vi "previewMovingBallIntercept.vi"(7 "destino original":dbl[](array[numeric]), 8 "error in (no error)":errorcluster, 9 "Robot in":refnum<class "Robot.lvclass">, 10 "BallRef":refnum<class "Ball.lvclass">, 11 "KickToSkill in":refnum<class "KickToSkill.lvclass">) -> (0 "error out":errorcluster, 1 "estimated_intercep_point":dbl[](array[numeric]), 2 "heuristic":dbl, 3 "KickToSkill out":refnum<class "KickToSkill.lvclass">)   [LabVIEW 2023, in "KickToSkill.lvclass"]
uses:
  KickToSkill.lvclass
  Robot_class/Robot.lvclass
  C:/Users/ebert/Documents/codes/SSL/repo/SSL_AI/Object_class/Object.lvclass
  Ball_class/Ball.lvclass
  Object_class/Object.lvclass/Object.ctl
  Ball_class/Ball.lvclass/Ball.ctl
  <vilib>/Analysis/baseanly.llb/Unit Vector (DBL).vi
  <vilib>/Analysis/_algsub.llb/Real Vector Norm.vi
  Object_class/Read x.vi
  Object_class/Read y.vi
  Ball_class/Read v_x.vi
  Ball_class/Read v_y.vi
  KickToSkill.lvclass/KickToSkill.ctl
  <vilib>/Analysis/NI_AALPro.lvlib
  <vilib>/Analysis/NI_AALBase.lvlib
  Game_class/Game.lvclass
  <vilib>/Analysis/baseanly.llb/Real Dot Product.vi
panel:
  out "Waveform Chart":dbl(graph)
  out "Array":dbl[][](array[numeric])
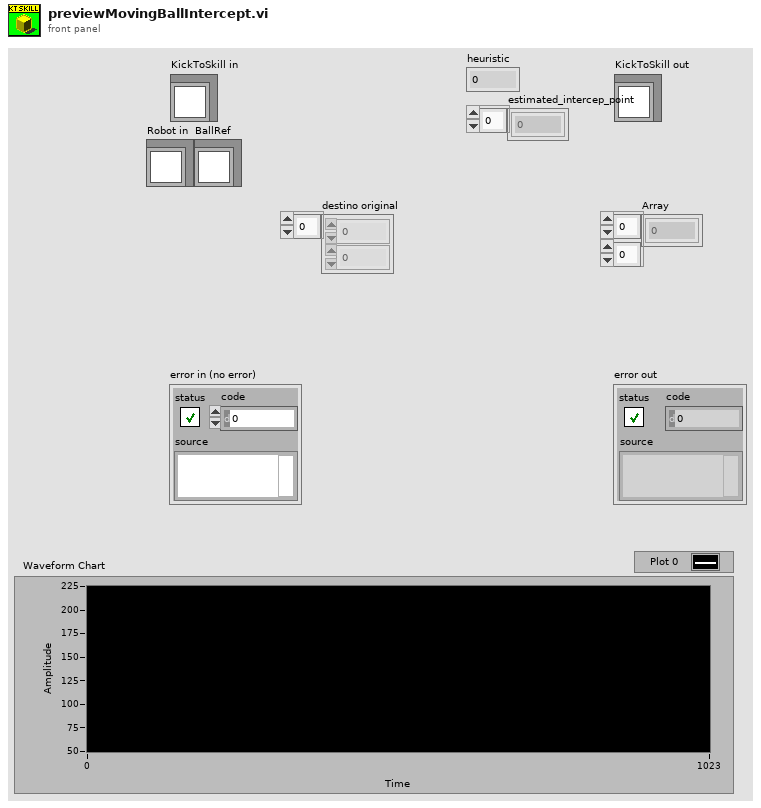
[diagram p1: front panel]
types:
  T1 = typedef "NI_Matrix.lvlib/RealMatrix.ctl" = dbl[][]
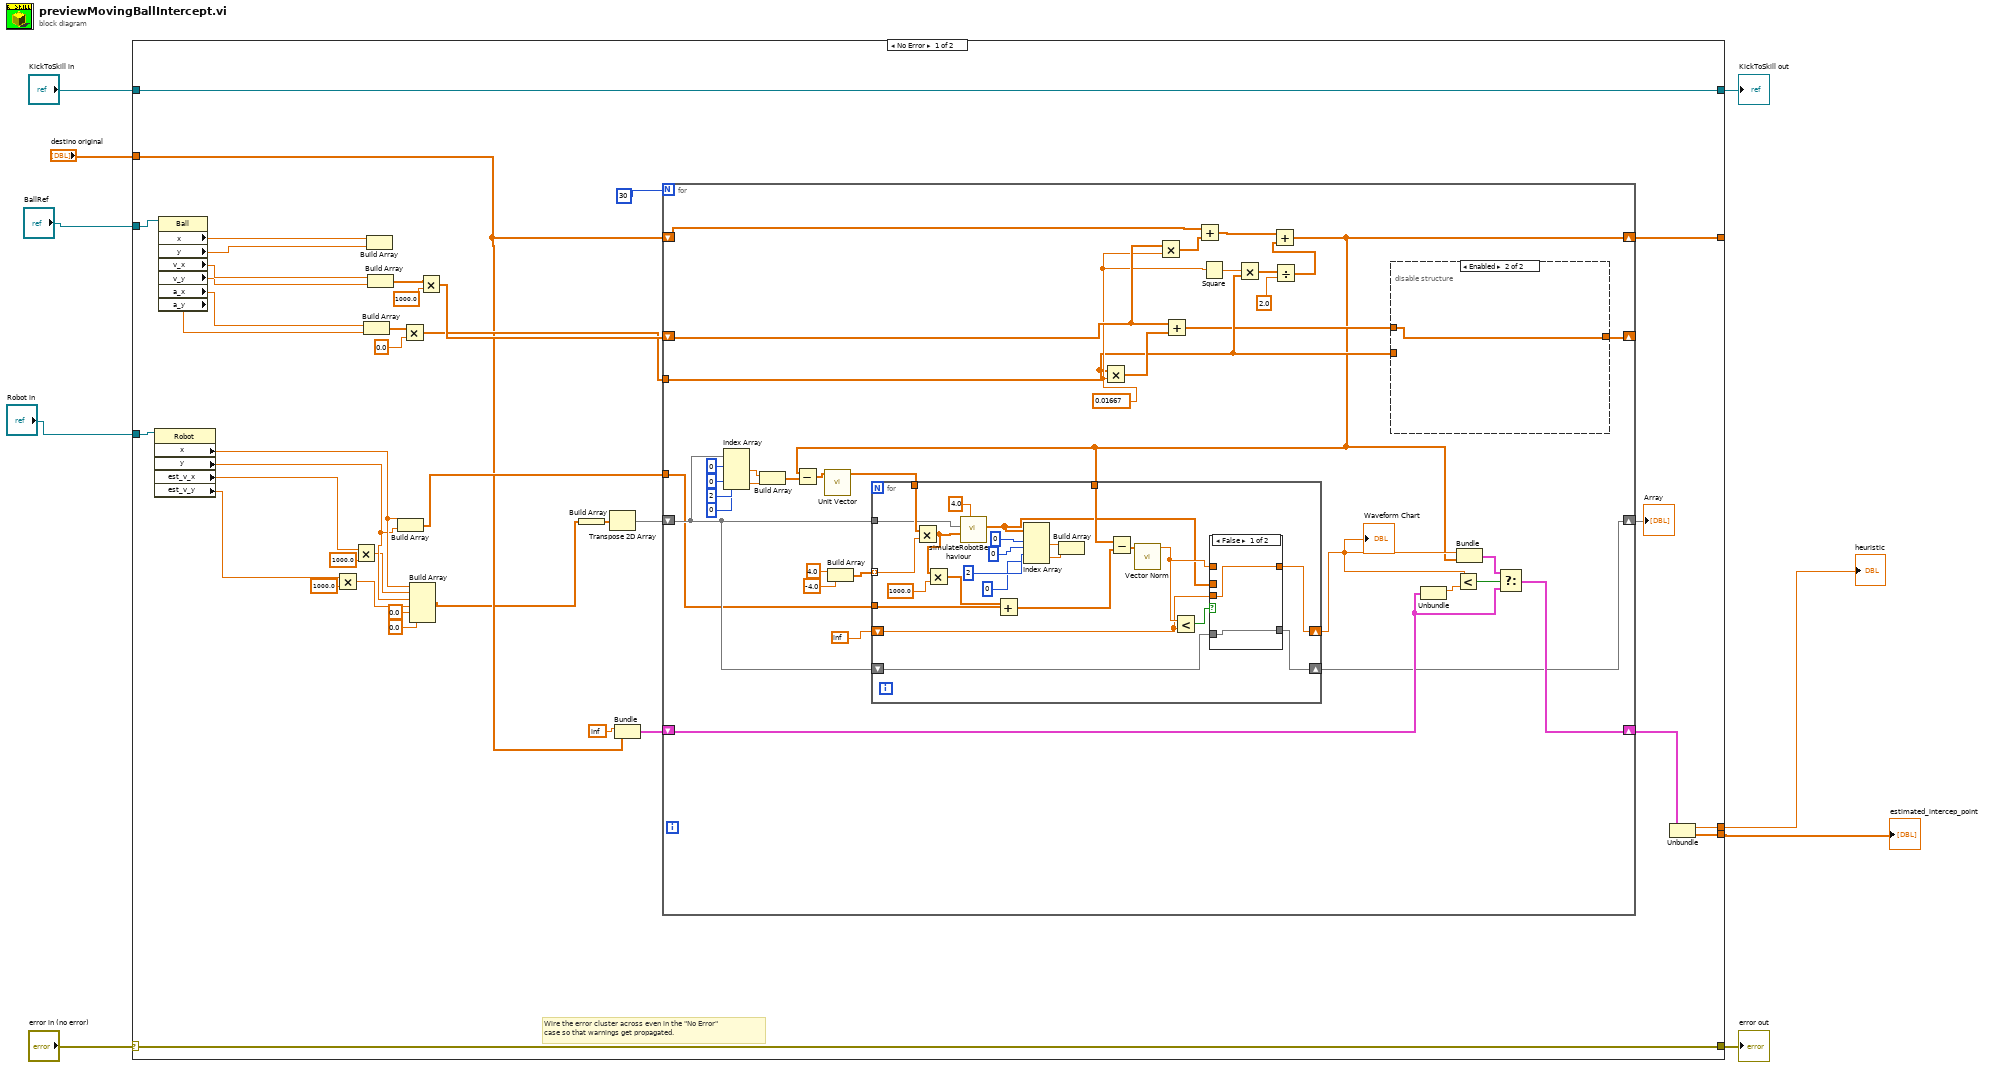
[diagram p0: block diagram]
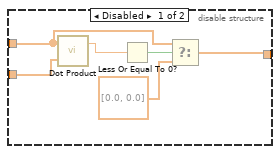
[diagram p3: hidden frame]
diagram:
  n1 = case shown="No Error" "error in (no error)" {
    selector: "error in (no error)" -> [w47 w121]
    tunnel: [w47 w121] -> w8
    tunnel: [w48 w120] -> w6
    tunnel: "KickToSkill in" -> [w48 w120]
    tunnel: "BallRef" -> [w44 _]
    tunnel: "Robot in" -> [w39 _]
    tunnel: [w36 _] -> w5
    tunnel: [w10 _] -> w4
    tunnel: [w11 _] -> _
    tunnel: "destino original" -> [w21 _]
    frame No Error {
      # "Wire the error cluster across even in the \"No Error\"\ncase so that warnings get propagated."
      n2 = property class="Robot"(reference=w39) -> ("x"=w27:dbl, "y"=w26:dbl, "est_v_x"=w16:dbl, "est_v_y"=w14:dbl)  [unwired: 1 in, 2 out]
      n3 = property class="Ball"(reference=w44) -> ("x"=w43:dbl, "y"=w42:dbl, "v_x"=w41:dbl, "v_y"=w40:dbl, "a_x"=w32:dbl, "a_y"=w31:dbl)  [unwired: 1 in, 2 out]
      n4 = Multiply(x=w14, y=1000.0) -> (x*y=w13:dbl)
      n5 = Multiply(x=w16, y=1000.0) -> (x*y=w15:dbl)
      n6 = Build Array(w32, w31) -> (w29:dbl[])
      n7 = Build Array(w43, w42) -> ()  [unwired: 1 out]
      n8 = Build Array(w41, w40) -> (w35:dbl[])
      n9 = Build Array(w27, w26) -> (w38:dbl[])
      n10 = Multiply(x=w29, y=0.0) -> (x*y=w28:dbl[])
      n11 = Build Array(w27, w15, w26, w13, 0.0 ("element"), 0.0 ("element")) -> (w19:dbl[])
      n12 = Multiply(x=w35, y=1000.0) -> (x*y=w33:dbl[])
      n13 = Build Array(w19) -> (w23:dbl[][])
      n14 = Transpose 2D Array(2D array=w23) -> (transposed array=w22:dbl[][])
      n15 = Bundle(inf, "destino original"=w21) -> (w45:cluster{dbl, "destino original":dbl[]})  [unwired: 1 in]
      n16 = for {
        N: 30 -> [_]
        tunnel: w28 -> [w75]
        shift-right: [w74] -> _
        shift-left: w33 -> [w84]
        shift-right: [w53] -> w11
        shift-left: w21 -> [w65]
        shift-right: [w71] -> w37
        shift-left: w45 -> [w72]
        tunnel: w38 -> [w49]
        shift-right: [w54] -> w20
        shift-left: w22 -> [w62]
        w81 = 0.01667 ("y")
        n17 = Index Array(array=w62, index (row) #1=0 ("index (row)"), index (col) #1=0 ("disabled index (col)"), index (row) #2=2 ("index (row)"), index (col) #2=0 ("disabled index (col)")) -> (element #1=w61:dbl, element #2=w60:dbl)
        n18 = Build Array(w61, w60) -> (w55:dbl[])
        n19 = Build Array(4.0 ("element"), -4.0 ("element")) -> (w50:dbl[])
        n20 = Multiply(x=w75, y=w81) -> (x*y=w79:dbl[])
        n21 = Multiply(x=w84, y=w81) -> (x*y=w83:dbl[])
        n22 = Add(x=w84, y=w79) -> (x+y=w73:dbl[])
        n23 = Add(x=w65, y=w83) -> (x+y=w82:dbl[])
        n24 = Square(x=w81) -> (x^2=w80:dbl)
        n25 = Multiply(x=w80, y=w75) -> (x*y=w78:dbl[])
        n26 = Divide(x=w78, y=2.0) -> (x/y=w76:dbl[])
        n27 = Add(x=w82, y=w76) -> (x+y=w53:dbl[])
        n28 = Subtract(x=w53, y=w55) -> (x-y=w67:dbl[])
        n29 = call-poly <vilib>:"Unit Vector.vi"("Input Vector"=w67) -> ("Unit Vector"=w66:dbl[])  [unwired: 8 in, 2 out]
        n30 = for {
          tunnel: w66 -> [w101]
          tunnel: w62 -> [w100]
          tunnel: w53 -> [w99]
          tunnel: w50 -> [w90] mode=indexing
          shift-right: [w96] -> w63
          shift-left: inf -> [w92]
          shift-right: [w93] -> w54
          shift-left: w62 -> [w95]
          tunnel: w49 -> [w89]
          n31 = Multiply(x=w101, y=w90) -> (x*y=w88:dbl[])
          n32 = Multiply(x=w88, y=1000.0) -> (x*y=w86:dbl[])
          n33 = call "simulateRobotBehaviour.vi"("max_accel"=4.0, "u_k"=w88, "x_k_k"=w100) -> ("x_k+1"=w94:T1)  [unwired: 6 in, 2 out]
          n34 = Add(x=w86, y=w89) -> (x+y=w85:dbl[])
          n35 = Index Array(array=w94, index (row) #1=0 ("index (row)"), index (col) #1=0 ("disabled index (col)"), index (row) #2=2 ("index (row)"), index (col) #2=0 ("disabled index (col)")) -> (element #1=w104:dbl, element #2=w103:dbl)
          n36 = Build Array(w104, w103) -> ()  [unwired: 1 out]
          n37 = Subtract(x=w99, y=w85) -> (x-y=w108:dbl[])
          n38 = call-poly <vilib>:"Vector Norm.vi"("Input Vector"=w108) -> ("norm"=w97:dbl)  [unwired: 9 in, 1 out]
          n39 = Less?(x=w97, y=w92) -> (x < y?=w98:bool)
          n40 = case shown="False" w98 {
            tunnel: w97 -> [_ w112]
            tunnel: [w109 w112] -> w96
            tunnel: w95 -> [w110 _]
            tunnel: w94 -> [_ w111]
            tunnel: [w110 w111] -> w93
            tunnel: w92 -> [w109 _]
            frame False {
            }
            frame True {
            }
          }
        }
        "Waveform Chart" <- w63
        n41 = disable-structure shown="Enabled" {
          disable-tunnel: w75 -> [w118 _]
          disable-tunnel: [w113 w119] -> w74
          disable-tunnel: w73 -> [w115 w119]
          frame Disabled {
            n42 = call-poly <vilib>:"Dot Product.vi"("Y Vector"=w118, "X Vector"=w115) -> ("X * Y"=w117:dbl)  [unwired: 1 out]
            n43 = Less Or Equal To 0?(x=w117) -> (x <= 0?=w116:bool)
            n44 = Select(t=w115, s=w116, f=dbl[] [0.0, 0.0]) -> (s? t:f=w113:dbl[])
          }
          frame Enabled {
          }
        }
        n45 = Unbundle(w72) -> (w70:dbl)  [unwired: 1 out]
        n46 = Less?(x=w63, y=w70) -> (x < y?=w69:bool)
        n47 = Bundle(w63, w53) -> (w68:cluster{dbl, dbl[]})  [unwired: 1 in]
        n48 = Select(t=w68, s=w69, f=w72) -> (s? t:f=w71:cluster{dbl, "destino original":dbl[]})
      }
      "Array" <- w20
      n49 = Unbundle(w37) -> (w36:dbl, "destino original"=w10:dbl[])
    }
    frame Error {
    }
  }
  "error out" <- w8
  "KickToSkill out" <- w6
  "heuristic" <- w5
  "estimated_intercep_point" <- w4
